vi "ColorToFXP.vi"(11 "Color (U64)":T1) -> (3 "Numeric":fxp<+,3,3>)   [LabVIEW 2019, in "RT_Game.lvlib" / "Game.lvclass"]
uses:
  Game.lvclass
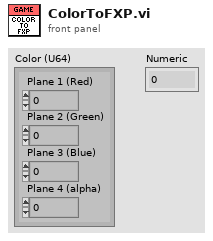
[diagram p1: front panel]
types:
  T1 = typedef "Color (U64)" = cluster{"Plane 3 (Blue)":u16, "Plane 2 (Green)":u16, "Plane 1 (Red)":u16, "Plane 4 (alpha)":u16}
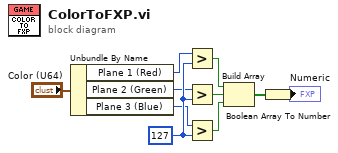
[diagram p0: block diagram]
diagram:
  w5 = u8 127 ("y")
  n1 = Unbundle By Name("Color (U64)") -> ("Plane 1 (Red)"=w2:u16, "Plane 2 (Green)"=w3:u16, "Plane 3 (Blue)"=w4:u16)
  n2 = Greater?(x=w2, y=w5) -> (0:w8:bool)
  n3 = Greater?(x=w3, y=w5) -> (0:w9:bool)
  n4 = Greater?(x=w4, y=w5) -> (0:w10:bool)
  n5 = Build Array(w8, w9, w10) -> (w6:bool[])
  n6 = Boolean Array To Number(Boolean array=w6) -> (number=→"Numeric":fxp<+,3,3>)
